vi "Read Measurement Data (Unit NChan).vi"(0 "VISA resource name":refnum<visa-resource-name>, 5 "Start Channel (1)":string="0001", 7 "End Channel (1)":string="0001", 11 "error in (no error)":errorcluster) -> (4 "VISA resource name out":refnum<visa-resource-name>, 6 "Channel":string[](array[string]), 10 "Data Status":i32[](array[ring]) items=["Normal", "Differential Input", "Skip"], 13 "Decimal Position":i32[](array[numeric]) max=4 step=1, 14 "Unit":string[](array[string]), 15 "error out":errorcluster)   [LabVIEW 2020, in "Yokogawa GX Series.lvlib"]
doc: "This VI reads the channel number, data status, decimal position, and unit."
uses:
  <instrlib>/Yokogawa GX Series/Yokogawa GX Series.lvlib
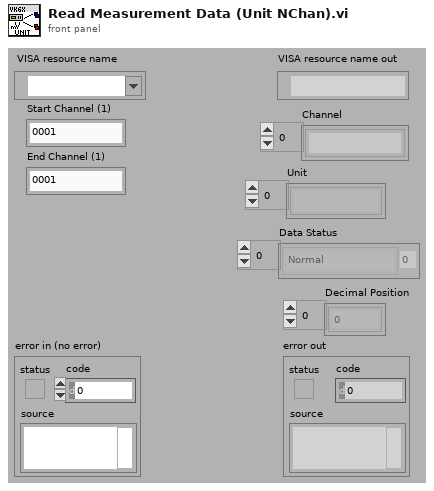
[diagram p1: front panel]
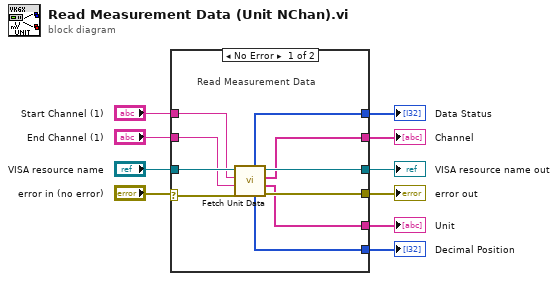
[diagram p0: block diagram]
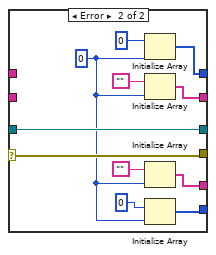
[diagram p2: hidden frame]
diagram:
  n1 = case shown="No Error" "error in (no error)" {
    selector: "error in (no error)" -> [w11 w30]
    tunnel: "VISA resource name" -> [w20 w31]
    tunnel: [w19 w31] -> w9
    tunnel: [w18 w30] -> w8
    tunnel: "Start Channel (1)" -> [w17 _]
    tunnel: "End Channel (1)" -> [w16 _]
    tunnel: [w15 w26] -> w5
    tunnel: [w14 w27] -> w4
    tunnel: [w13 w22] -> w3
    tunnel: [w12 w25] -> w2
    frame No Error {
      # "Read Measurement Data"
      n2 = call <instrlib>:"Fetch Unit Data.vi"("error in (no error)"=w11, "End Channel (1)"=w16, "Start Channel (1)"=w17, "VISA resource name"=w20) -> ("error out"=w18:errorcluster, "Unit"=w12:string[], "Channel"=w15:string[], "VISA resource name out"=w19:refnum<visa-resource-name>, "Decimal Position"=w13:i32[], "Data Status"=w14:i32[])  [unwired: 2 out]
    }
    frame Error {
      w21 = 0
      n3 = Initialize Array(0, w21) -> (w27:i32[])
      n4 = Initialize Array("", w21) -> (w26:string[])
      n5 = Initialize Array("", w21) -> (w25:string[])
      n6 = Initialize Array(0, w21) -> (w22:i32[])
    }
  }
  "error out" <- w8
  "VISA resource name out" <- w9
  "Unit" <- w2
  "Data Status" <- w4
  "Channel" <- w5
  "Decimal Position" <- w3
